vi "set pixel.vi"(8 "error in (no error)":errorcluster, 9 "dummy":u16, 10 "davalue":u16, 11 "pulswidth":u16) -> (0 "error out":errorcluster)   [LabVIEW 2015, in "SCANalone4x64.lvlib"]
doc: "__declspec(dllimport) void __stdcall set_pixel(unsigned short pulswidth, unsigned short davalue, unsigned short dummy);"
uses:
  <userlib>/SCANalone4x64/SCANalone4x64.lvlib
  <userlib>/SCANalone4x64/SCANalone4x64.dll
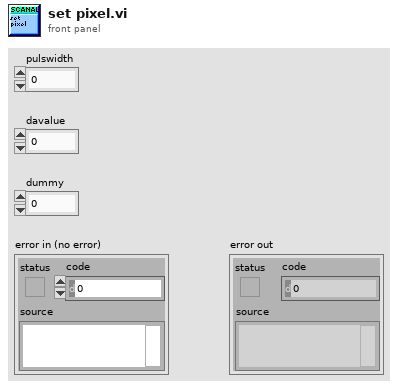
[diagram p1: front panel]
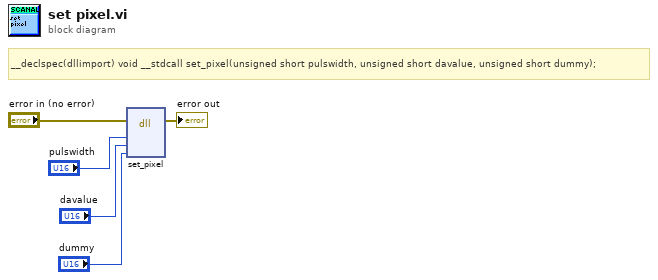
[diagram p0: block diagram]
diagram:
  # "__declspec(dllimport) void __stdcall set_pixel(unsigned short pulswidth, unsigned short davalue, unsigned short dummy);"
  n1 = dll-call lib="C:/Program Files/National Instruments/LabVIEW 2015/user.lib/SCANalone4x64/SCANalone4x64.*" fn="set_pixel"(error in="error in (no error)", "pulswidth"="pulswidth", "davalue"="davalue", "dummy"="dummy") -> (error out=→"error out":errorcluster)  [unwired: 6 in, 1 out]
